vi "Verify Drum and Heater Relays.vi"(5 "Expected Relay State":T1, 7 "Care":T1, 11 "Error In":errorcluster) -> (4 "Pass/Fail":bool, 6 "Actual Relay State":T1, 8 "Report Text":string, 15 "Error Out":errorcluster)   [LabVIEW 2016]
uses:
  TypeDefs/Drum and Heater Relay State.ctl
  <vilib>/DAQmx/read.llb/DAQmx Read (Digital 1D Bool NChan 1Samp 1Line).vi
  <vilib>/DAQmx/create/channels.llb/DAQmx Create Channel (DI-Digital Input).vi
  <vilib>/DAQmx/miscellaneous.llb/DAQmx Fill In Error Info.vi
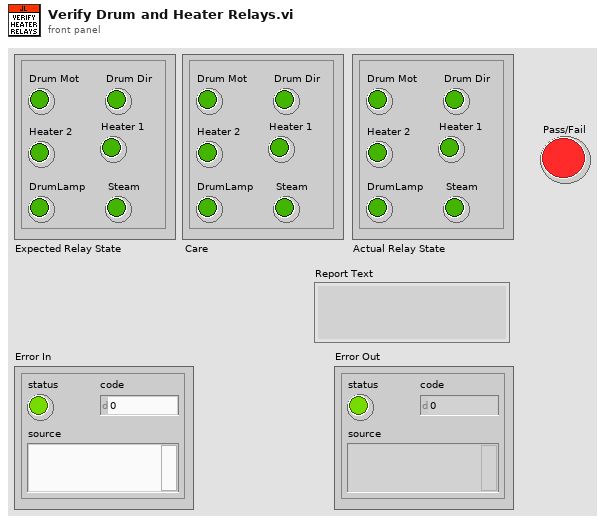
[diagram p1: front panel]
types:
  T1 = typedef "Drum and Heater Relay State.ctl" = cluster{"Steam":bool, "Drum Mot":bool, "Drum Dir":bool, "Heater 1":bool, "Heater 2":bool, "DrumLamp":bool}
  T2 = cluster{"data[0]":bool, "data[1]":bool, "data[2]":bool, "data[3]":bool, "data[4]":bool, "data[5]":bool}
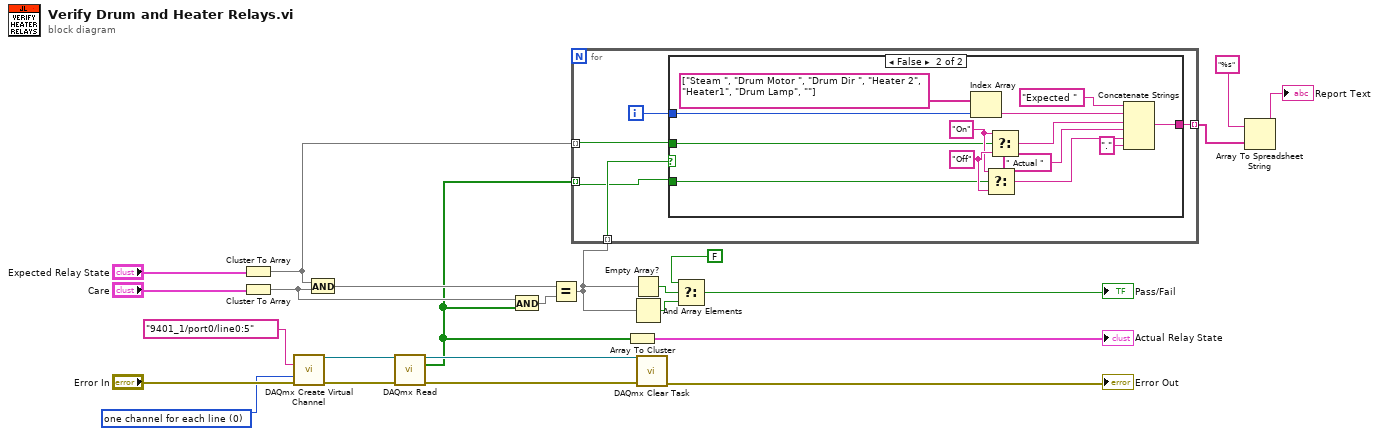
[diagram p0: block diagram]
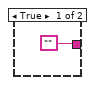
[diagram p2: hidden frame]
diagram:
  w10 = 0 items=["one channel for each line", "one channel for all lines"] ("line grouping")
  n1 = Cluster To Array(cluster="Expected Relay State") -> (array=w8:bool[])
  n2 = Cluster To Array(cluster="Care") -> (array=w18:bool[])
  n3 = call-poly <vilib>:"DAQmx Create Virtual Channel.vi"("lines"=tag "9401_1/port0/line0:5", "line grouping"=w10, "error in"="Error In") -> ("task out"=w23:refnum<k21>, "error out"=w22:errorcluster)  [unwired: 11 in]
  n4 = And(x=w8, y=w18) -> (x .and. y?=w9:bool[])
  n5 = call-poly <vilib>:"DAQmx Read.vi"("task/channels in"=w23, "error in"=w22) -> ("task out"=w21:refnum<k21>, "data"=w1:bool[], "error out"=w20:errorcluster)  [unwired: 11 in]
  n6 = And(x=w18, y=w1) -> (x .and. y?=w17:bool[])
  n7 = Equal?(x=w9, y=w17) -> (x = y?=w7:bool[])
  n8 = for {
    tunnel: w8 -> [w25] mode=indexing
    tunnel: w1 -> [w26] mode=indexing
    tunnel: [w29] -> w4 mode=indexing
    tunnel: w7 -> [w28] mode=indexing
    i -> [w27]
    n9 = case shown="False" w28 {
      tunnel: w25 -> [_ w38]
      tunnel: w26 -> [_ w37]
      tunnel: ["" w34] -> w29
      tunnel: w27 -> [_ w31]
      frame True {
      }
      frame False {
        w40 = "Off"
        w39 = "On"
        n10 = Index Array(array=string[] ["Steam ", "Drum Motor ", "Drum Dir ", "Heater 2", "Heater1", "Drum Lamp", ""], index=w31) -> (element=w32:string)
        n11 = Select(t=w39, s=w37, f=w40) -> (s? t:f=w36:string)
        n12 = Select(t=w39, s=w38, f=w40) -> (s? t:f=w42:string)
        n13 = Concatenate Strings("Expected " ("string"), w32, w42, " Actual " ("string"), w36, "." ("string")) -> (w34:string)
      }
    }
  }
  n14 = Array To Cluster(array=w1) -> (cluster=→"Actual Relay State":T2)
  n15 = Empty Array?(array=w7) -> (empty?=w14:bool)
  n16 = And Array Elements(Boolean array=w7) -> (logical AND=w16:bool)
  n17 = call <vilib>:"DAQmx Clear Task.vi"("task in"=w21, "error in"=w20) -> ("error out"=→"Error Out":errorcluster)  [unwired: 13 in]
  n18 = Select(t=FALSE, s=w14, f=w16) -> (s? t:f=→"Pass/Fail":bool)
  n19 = Array To Spreadsheet String(array=w4, 3:"%s" ("delimiter (Tab)")) -> (spreadsheet string=→"Report Text":string)  [unwired: 1 in]
